vi "licdf record write.vi"(7 "data_len":i32, 8 "error in (no error)":errorcluster, 9 "data":string, 10 "name":string, 11 "handle":i32) -> (0 "error out":errorcluster, 3 "function return":i32)   [LabVIEW 2026, in "keynub_licdongle.lvlib"]
doc: "int32_t licdf_record_write(int32_t handle, const char *name, const uint8_t *data,\n int32_t data_len);"
uses:
  keynub_licdongle.lvlib
  natives/win-x64/keynub_licdongle_flat.dll
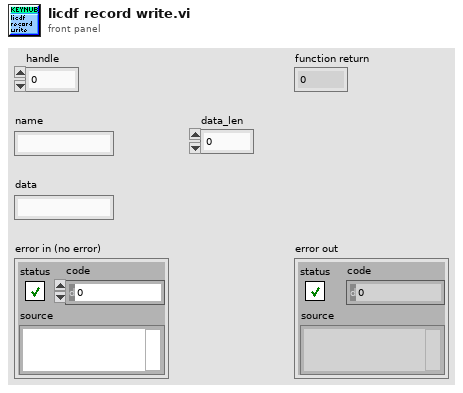
[diagram p1: front panel]
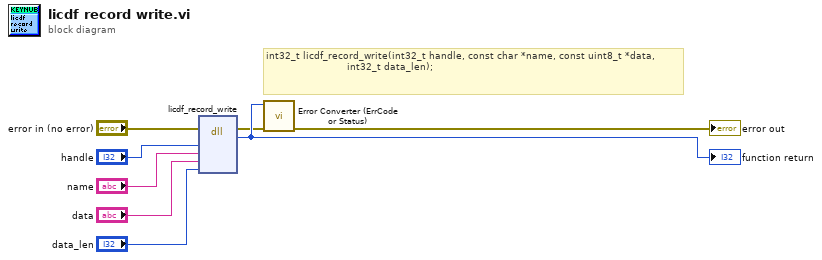
[diagram p0: block diagram]
diagram:
  # "int32_t licdf_record_write(int32_t handle, const char *name, const uint8_t *data,\n                           int32_t data_len);"
  n1 = dll-call lib="C:/Austausch/KeyNub/LicenseDongle-PublicSDK/natives/win-x64/keynub_licdongle_flat.*" fn="licdf_record_write"(error in="error in (no error)", "handle"="handle", "name"="name", "data"="data", "data_len"="data_len") -> (error out=w2:errorcluster, w8:i32)  [unwired: 6 in, 1 out]
  "function return" <- w8
  n2 = call "Error Converter (ErrCode or Status).vi"("error in (no error)"=w2, "error code"=w8) -> ("error out"=→"error out":errorcluster)  [unwired: 9 in]
